vi "Send Local Message.vi"(0 "message queue in":T2, 1 "receiver process (\"\" - local)":string, 5 "message name":string, 7 "message value":string, 9 "timeout (-1 ms)":i32=-1, 11 "error in":errorcluster, 12 "message attributes":T1, 13 "priority message (F)":bool) -> (4 "message queue out":T2, 10 "timed out?":bool, 15 "error out":errorcluster)   [LabVIEW 2015, in "TLB` Template.lvlib" / "AMC.lvlib"]
doc: "Adds a message to the local message queue provided by the queue reference or to another message queue in the local application based on the receiver process name.\n\nIf \"priority message\" is True, the message will be added to the front of the message queue.TLB Prime - Application Template 1.3.0.24\nNorm Kirchner, NI Systems Engineering - NI\nCopyright (c) 2014, NI"
uses:
  AMC.lvlib
  Message Queue.ctl
  Message.ctl
  KeyedArray.ctl
  Tools_KeyedArray.lvlib
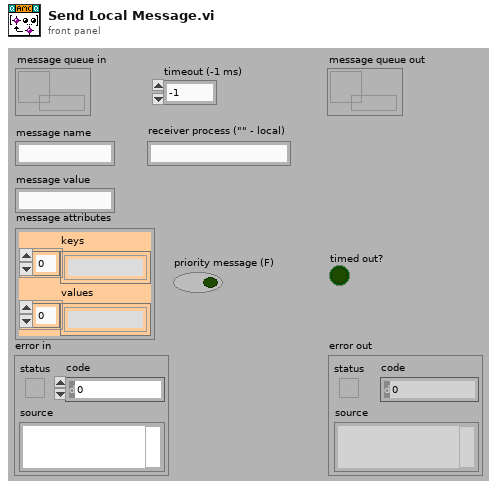
[diagram p1: front panel]
types:
  T1 = typedef "TLB` Template.lvlib/Tools_KeyedArray.lvlib/KeyedArray.ctl" = cluster{"keys":string[], "values":string[]}
  T2 = typedef "TLB` Template.lvlib/AMC.lvlib/Message Queue.ctl" = refnum<queue>
  T3 = typedef "TLB` Template.lvlib/AMC.lvlib/Message.ctl" = cluster{"name":string, "value":string, "attributes":T1, "receiver host":string, "receiver process":string, "source host":string, "source process":string, "priority message":bool, "acknowledge message":bool}
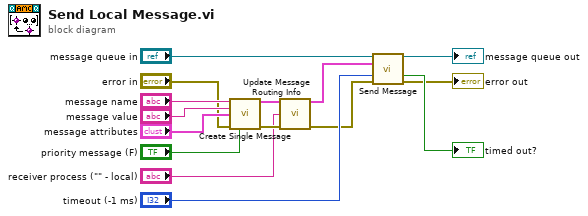
[diagram p0: block diagram]
diagram:
  n1 = call "Create Single Message.vi"("name"="message name", "value"="message value", "attributes"="message attributes", "error in"="error in", "priority message (F)"="priority message (F)") -> ("message"=w6:T3, "error out"=w4:errorcluster)  [unwired: 9 in]
  n2 = call "Update Message Routing Info.vi"("message"=w6, "receiver process (\"\")"="receiver process (\"\" - local)", "error in"=w4) -> ("message"=w5:T3, "error out"=w2:errorcluster)  [unwired: 11 in]
  n3 = call "Send Message.vi"("message queue in"="message queue in", "message"=w5, "timeout (-1 ms)"="timeout (-1 ms)", "error in"=w2) -> ("message queue out"=→"message queue out":T2, "timed out?"=→"timed out?":bool, "error out"=→"error out":errorcluster)  [unwired: 9 in]
